vi "GetAccumulatorDeviceConstants.vi"(11 "key values":T1[](array[typedef])) -> (1 "default data block length (sec)":dbl, 2 "min block (sec)":dbl, 3 "max block (sec)":dbl, 5 "max low rate memory (percent)":dbl, 7 "max low rate cpu (percent)":dbl)   [LabVIEW 2017, in "DataAccumulator.lvlib"]
uses:
  <vilib>/addons/InsightCM/Devices/Shared/Common/DataAccumulator/DataAccumulator.lvlib
  <vilib>/addons/InsightCM/MessageBus/Base/controls/SectionKeyValues.ctl
  <vilib>/addons/InsightCM/MessageBus/Base/controls/KeyValuePair.ctl
  <vilib>/addons/InsightCM/Utilities/PropertyHelpers/PropertyHelpers.lvlib
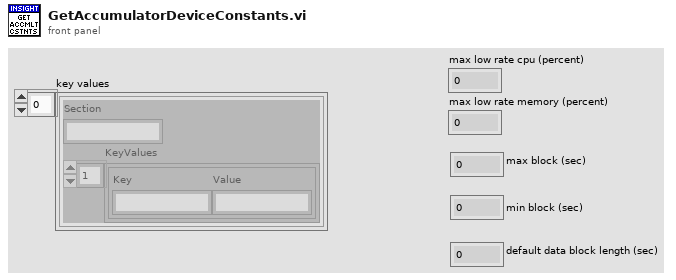
[diagram p1: front panel]
types:
  T1 = typedef "SectionKeyValues.ctl" = cluster{"Section":string, "KeyValues":T2[]}
  T2 = typedef "KeyValuePair.ctl" = cluster{"Key":string, "Value":string}
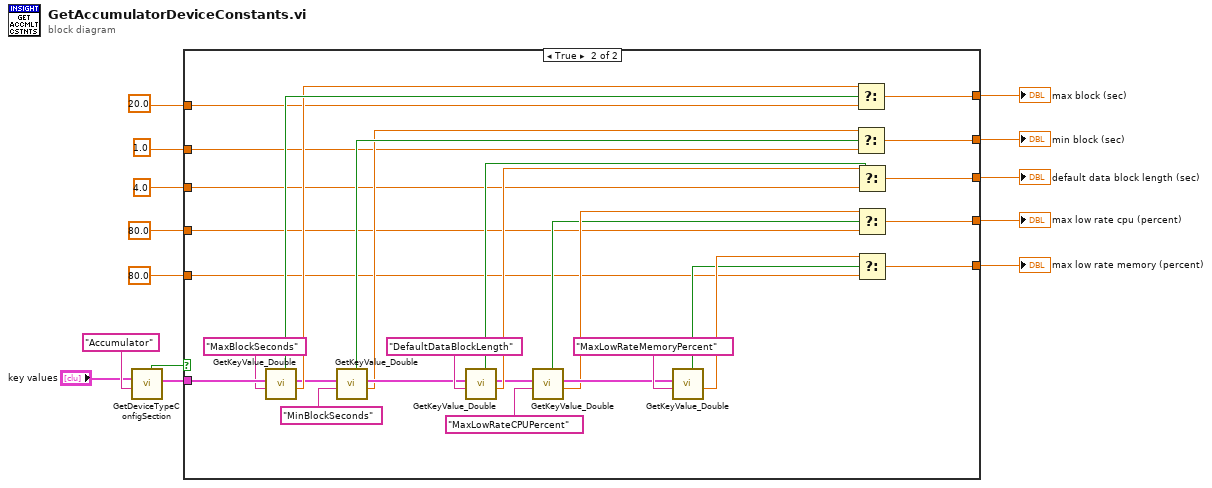
[diagram p0: block diagram]
diagram:
  n1 = call <vilib>:"GetDeviceTypeConfigSection.vi"("key"="Accumulator", "key values"="key values") -> ("key value pairs out"=w11:T2[], "found"=w12:bool)  [unwired: 8 in]
  n2 = case shown="True" w12 {
    tunnel: w11 -> [_ w49]
    tunnel: [w19 w37] -> w10
    tunnel: [w18 w36] -> w9
    tunnel: [w17 w31] -> w8
    tunnel: [w16 w29] -> w7
    tunnel: [w15 w30] -> w6
    tunnel: 20.0 ("f") -> [w19 w24]
    tunnel: 1.0 ("f") -> [w18 w23]
    tunnel: 4.0 ("f") -> [w17 w22]
    tunnel: 80.0 ("f") -> [w16 w21]
    tunnel: 80.0 ("f") -> [w15 w20]
    frame False {
    }
    frame True {
      n3 = call <vilib>:"GetKeyValue_Double.vi"("key"="MaxBlockSeconds" ("Key"), "key value pairs"=w49) -> ("value"=w47:dbl, "key value pairs out"=w44:T2[], "found"=w48:bool)  [unwired: 7 in]
      n4 = call <vilib>:"GetKeyValue_Double.vi"("key"="MinBlockSeconds" ("Key"), "key value pairs"=w44) -> ("value"=w38:dbl, "key value pairs out"=w42:T2[], "found"=w41:bool)  [unwired: 7 in]
      n5 = call <vilib>:"GetKeyValue_Double.vi"("key"="DefaultDataBlockLength" ("Key"), "key value pairs"=w42) -> ("value"=w39:dbl, "key value pairs out"=w33:T2[], "found"=w40:bool)  [unwired: 7 in]
      n6 = call <vilib>:"GetKeyValue_Double.vi"("key"="MaxLowRateCPUPercent" ("Key"), "key value pairs"=w33) -> ("value"=w28:dbl, "key value pairs out"=w32:T2[], "found"=w27:bool)  [unwired: 7 in]
      n7 = call <vilib>:"GetKeyValue_Double.vi"("key"="MaxLowRateMemoryPercent" ("Key"), "key value pairs"=w32) -> ("value"=w26:dbl, "found"=w25:bool)  [unwired: 7 in, 1 out]
      n8 = Select(t=w47, s=w48, f=w24) -> (s? t:f=w37:dbl)
      n9 = Select(t=w38, s=w41, f=w23) -> (s? t:f=w36:dbl)
      n10 = Select(t=w39, s=w40, f=w22) -> (s? t:f=w31:dbl)
      n11 = Select(t=w28, s=w27, f=w21) -> (s? t:f=w29:dbl)
      n12 = Select(t=w26, s=w25, f=w20) -> (s? t:f=w30:dbl)
    }
  }
  "max block (sec)" <- w10
  "min block (sec)" <- w9
  "default data block length (sec)" <- w8
  "max low rate cpu (percent)" <- w7
  "max low rate memory (percent)" <- w6
